vi "HasRectIntersectionFloat.vi"(8 "No Error":errorcluster, 10 "B":T1, 11 "A":T1) -> (0 "Error Out":errorcluster, 3 "Intersect?":bool)   [LabVIEW 2024, in "SDL3.lvlib" / "Rect.lvlib"]
doc: "<B>Summary</B>\nDetermine whether two rectangles intersect with float precision."
uses:
  Rect.lvlib
  Lib/SDL3.dll
  FRect--cluster.ctl
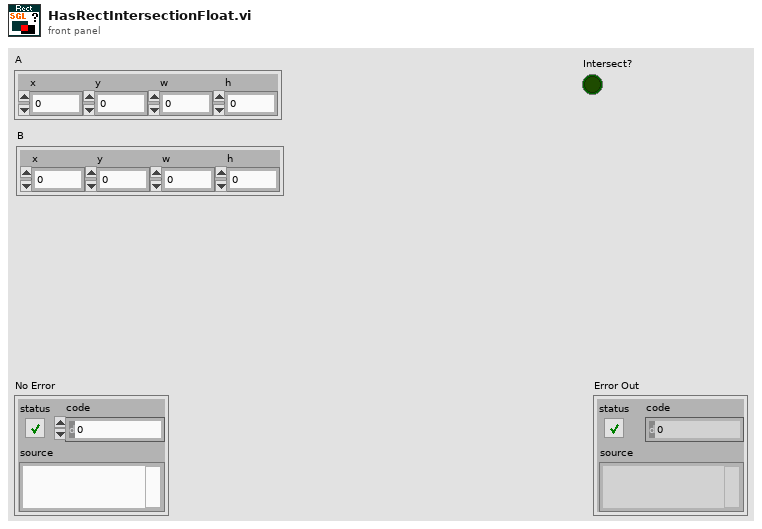
[diagram p1: front panel]
types:
  T1 = typedef "SDL3.lvlib/Rect.lvlib/FRect--cluster.ctl" = cluster{"x":sgl, "y":sgl, "w":sgl, "h":sgl}
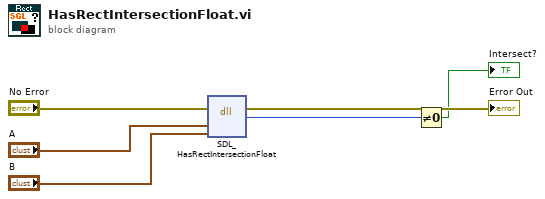
[diagram p0: block diagram]
diagram:
  n1 = dll-call lib="C:/Users/Thomas/Documents/Projects/LV-SDL3/Sources/SDL3/Lib/SDL3.*" fn="SDL_HasRectIntersectionFloat"(error in="No Error", "A"="A", "B"="B") -> (error out=→"Error Out":errorcluster, "return type"=w4:i32)  [unwired: 4 in, 1 out]
  n2 = Not Equal To 0?(x=w4) -> (x != 0?=→"Intersect?":bool)
